vi "GenerateAquatrakCalibrationSheet.vi"(11 "Data in":T1) -> (3 "Cal Sheet":string)   [LabVIEW 2018]
uses:
  <vilib>/Analysis/baseanly.llb/Mean (DBL).vi
  <vilib>/Analysis/NI_AALBase.lvlib
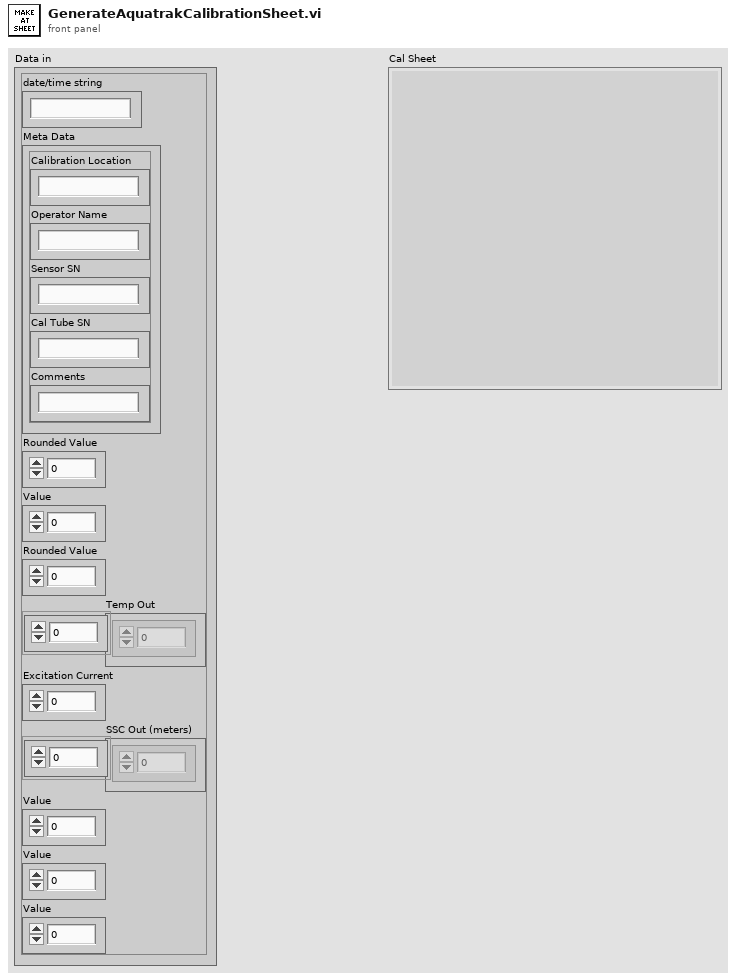
[diagram p1: front panel]
types:
  T1 = cluster{"date/time string":string, "Meta Data":cluster{"Calibration Location":string, "Operator Name":string, "Sensor SN":string, "Cal Tube SN":string, "Comments":string}, "Rounded Value":dbl, "Value":dbl, "Rounded Value":dbl, "Temp Out":dbl[], "Excitation Current":dbl, "SSC Out (meters)":dbl[], "Value":dbl, "Value":dbl, "Value":dbl}
  T2 = cluster{"Calibration Location":string, "Operator Name":string, "Sensor SN":string, "Cal Tube SN":string, "Comments":string}
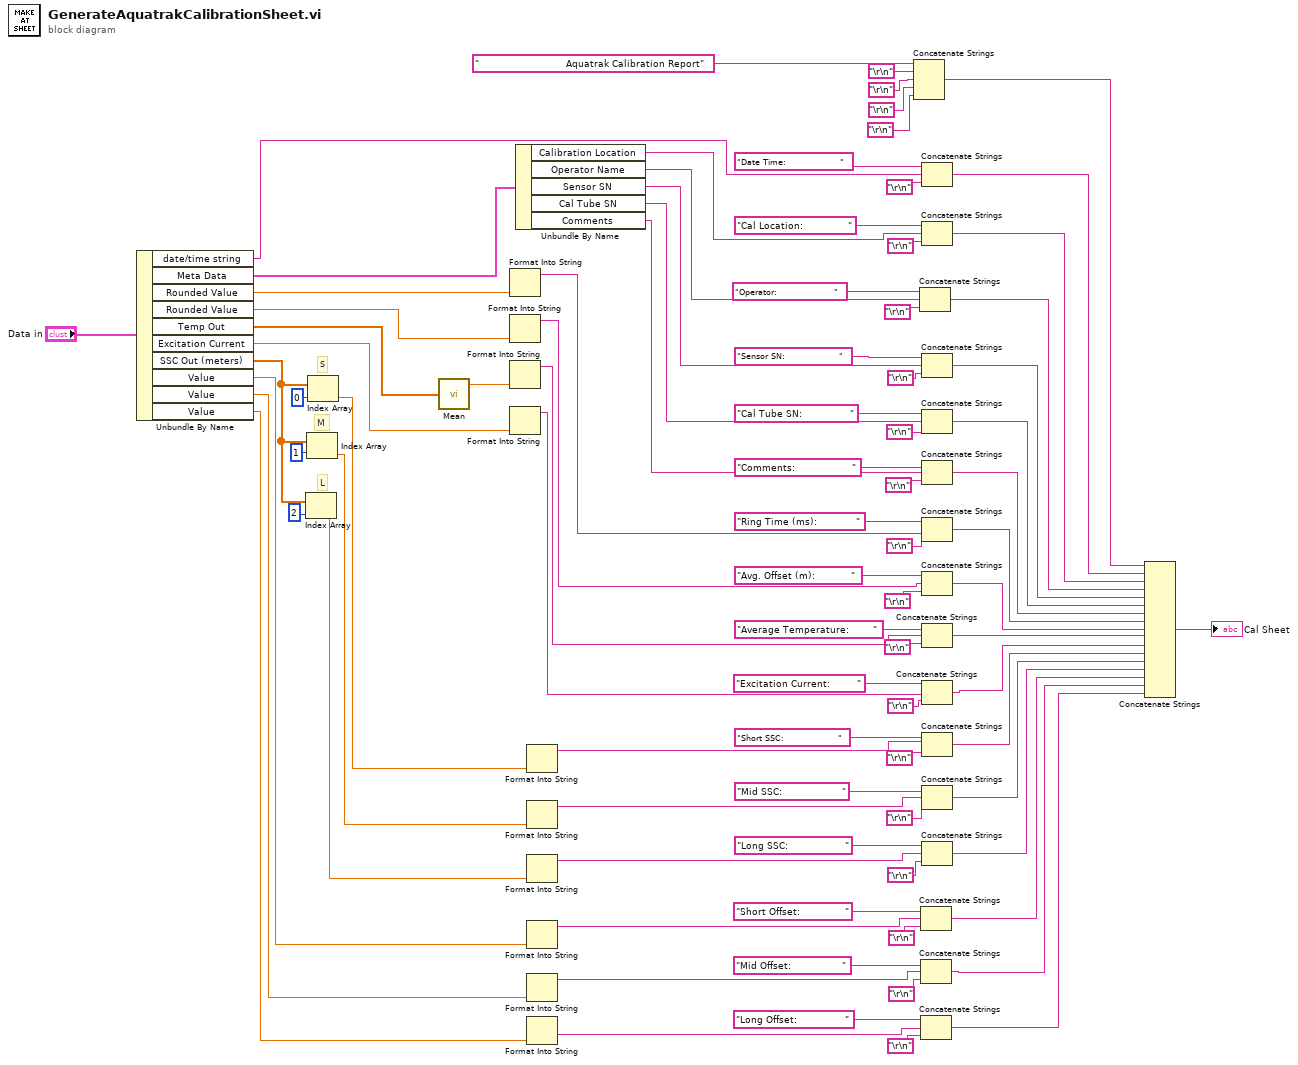
[diagram p0: block diagram]
diagram:
  # "L"
  # "M"
  # "S"
  n1 = Unbundle By Name("Data in") -> ("date/time string"=w19:string, "Meta Data"=w88:T2, "Rounded Value"=w65:dbl, "Rounded Value"=w26:dbl, "Temp Out"=w28:dbl[], "Excitation Current"=w29:dbl, "SSC Out (meters)"=w87:dbl[], "Value"=w45:dbl, "Value"=w46:dbl, "Value"=w47:dbl)
  n2 = Index Array(array=w87, index=2) -> (element=w33:dbl)
  n3 = Index Array(array=w87, index=1) -> (element=w34:dbl)
  n4 = Index Array(array=w87, index=0) -> (element=w35:dbl)
  n5 = call-poly <vilib>:"Mean.vi"("X"=w28) -> ("mean"=w27:dbl)  [unwired: 1 out]
  n6 = Format Into String(w65) -> (resulting string=w49:string)  [unwired: 3 in, 1 out]
  n7 = Format Into String(w26) -> (resulting string=w22:string)  [unwired: 3 in, 1 out]
  n8 = Format Into String(w27) -> (resulting string=w23:string)  [unwired: 3 in, 1 out]
  n9 = Format Into String(w29) -> (resulting string=w20:string)  [unwired: 3 in, 1 out]
  n10 = Unbundle By Name(w88) -> ("Calibration Location"=w60:string, "Operator Name"=w56:string, "Sensor SN"=w55:string, "Cal Tube SN"=w53:string, "Comments"=w51:string)
  n11 = Format Into String(w35) -> (resulting string=w32:string)  [unwired: 3 in, 1 out]
  n12 = Format Into String(w34) -> (resulting string=w31:string)  [unwired: 3 in, 1 out]
  n13 = Format Into String(w33) -> (resulting string=w30:string)  [unwired: 3 in, 1 out]
  n14 = Format Into String(w45) -> (resulting string=w36:string)  [unwired: 3 in, 1 out]
  n15 = Format Into String(w46) -> (resulting string=w37:string)  [unwired: 3 in, 1 out]
  n16 = Format Into String(w47) -> (resulting string=w38:string)  [unwired: 3 in, 1 out]
  n17 = Concatenate Strings("                             Aquatrak Calibration Report", "\r\n", "\r\n", "\r\n", "\r\n") -> (w66:string)
  n18 = Concatenate Strings("Operator:                   ", w56, "\r\n") -> (w15:string)
  n19 = Concatenate Strings("Short Offset:               ", w36, "\r\n") -> (w4:string)
  n20 = Concatenate Strings("Mid Offset:                 ", w37, "\r\n") -> (w3:string)
  n21 = Concatenate Strings("Long Offset:                ", w38, "\r\n") -> (w2:string)
  n22 = Concatenate Strings("Date Time:                  ", w19, "\r\n") -> (w17:string)
  n23 = Concatenate Strings("Cal Location:               ", w60, "\r\n") -> (w16:string)
  n24 = Concatenate Strings("Sensor SN:                  ", w55, "\r\n") -> (w14:string)
  n25 = Concatenate Strings("Cal Tube SN:                ", w53, "\r\n") -> (w13:string)
  n26 = Concatenate Strings("Comments:                   ", w51, "\r\n") -> (w12:string)
  n27 = Concatenate Strings("Ring Time (ms):             ", w49, "\r\n") -> (w11:string)
  n28 = Concatenate Strings("Avg. Offset (m):            ", w22, "\r\n") -> (w10:string)
  n29 = Concatenate Strings("Average Temperature:        ", w23, "\r\n") -> (w9:string)
  n30 = Concatenate Strings("Excitation Current:         ", w20, "\r\n") -> (w8:string)
  n31 = Concatenate Strings("Short SSC:                  ", w32, "\r\n") -> (w7:string)
  n32 = Concatenate Strings("Mid SSC:                    ", w31, "\r\n") -> (w6:string)
  n33 = Concatenate Strings("Long SSC:                   ", w30, "\r\n") -> (w5:string)
  n34 = Concatenate Strings(w66, w17, w16, w15, w14, w13, w12, w11, w10, w9, w8, w7, w6, w5, w4, w3, w2) -> (→"Cal Sheet":string)
